vi "EXCOM-TCP-26.vi"(0 "connection ID":refnum<k5>, 11 "Error IN":errorcluster) -> (2 "STATL":bool[](array[boolean])=[TRUE, FALSE, FALSE, FALSE, FALSE, FALSE, FALSE, FALSE, FALSE, FALSE, FALSE, FALSE, FALSE, FALSE, FALSE, FALSE, FALSE, FALSE, FALSE, FALSE, FALSE, FALSE, FALSE, FALSE, FALSE, FALSE, FALSE, FALSE, FALSE, FALSE, FALSE, FALSE], 3 "STATH":bool[](array[boolean])=[FALSE, FALSE, TRUE, TRUE, FALSE, TRUE, TRUE, FALSE, FALSE, FALSE, FALSE, FALSE, FALSE, FALSE, FALSE, FALSE, FALSE, FALSE, FALSE, FALSE, FALSE, FALSE, FALSE, FALSE, FALSE, FALSE, FALSE, FALSE, FALSE, FALSE, FALSE, FALSE], 4 "CID Out":refnum<k5>, 13 "STATEX":bool[](array[boolean]), 14 "STATLH":bool[](array[boolean]), 15 "Error Out":errorcluster)   [LabVIEW 2011]
panel:
  out "Response":string
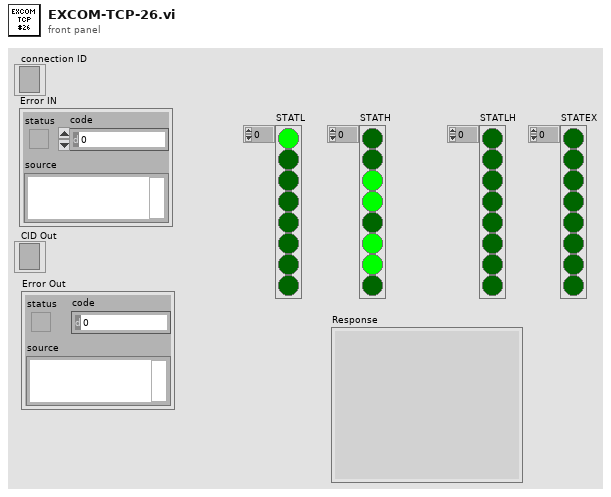
[diagram p1: front panel]
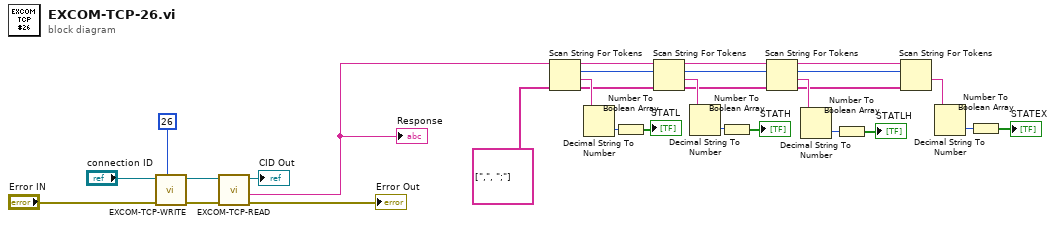
[diagram p0: block diagram]
diagram:
  w1 = string[] [",", ";"] ("delimiters (\\s,\\t,\\r,\\n)")
  n1 = call "EXCOM-TCP-WRITE.vi"("Commande #"=26, "Error IN"="Error IN", "connection ID"="connection ID") -> ("Error OUT"=w23:errorcluster, "connection ID out"=w24:refnum<k5>)  [unwired: 4 in, 2 out]
  n2 = call "EXCOM-TCP-READ.vi"("Error In"=w23, "connection ID"=w24) -> ("Error Out"=→"Error Out":errorcluster, "Response"=w2:string, "CID Out"=→"CID Out":refnum<k5>)  [unwired: 5 in]
  "Response" <- w2
  n3 = Scan String For Tokens(6:w1, 9:w2) -> (1:w8:string, 2:w6:i32, 3:w7:string)  [unwired: 4 in, 1 out]
  n4 = Decimal String To Number(string=w8) -> (number=w10:i32)  [unwired: 2 in, 1 out]
  n5 = Number To Boolean Array(number=w10) -> (Boolean array=→"STATL":bool[])
  n6 = Scan String For Tokens(6:w1, 8:w6, 9:w7) -> (1:w4:string, 2:w5:i32, 3:w3:string)  [unwired: 3 in, 1 out]
  n7 = Decimal String To Number(string=w4) -> (number=w12:i32)  [unwired: 2 in, 1 out]
  n8 = Number To Boolean Array(number=w12) -> (Boolean array=→"STATH":bool[])
  n9 = Scan String For Tokens(6:w1, 8:w5, 9:w3) -> (1:w9:string, 2:w18:i32, 3:w19:string)  [unwired: 3 in, 1 out]
  n10 = Decimal String To Number(string=w9) -> (number=w13:i32)  [unwired: 2 in, 1 out]
  n11 = Number To Boolean Array(number=w13) -> (Boolean array=→"STATLH":bool[])
  n12 = Scan String For Tokens(6:w1, 8:w18, 9:w19) -> (1:w16:string)  [unwired: 3 in, 3 out]
  n13 = Decimal String To Number(string=w16) -> (number=w17:i32)  [unwired: 2 in, 1 out]
  n14 = Number To Boolean Array(number=w17) -> (Boolean array=→"STATEX":bool[])
